vi "superactuator.vi"(8 "error in (no error)":errorcluster, 11 "BMC in":refnum<class "BMC.lvclass">) -> (0 "error out":errorcluster, 3 "BMC out":refnum<class "BMC.lvclass">)   [LabVIEW 2012, in "BMC.lvclass"]
uses:
  BMC.lvclass
  BMC.lvclass/BMC.ctl
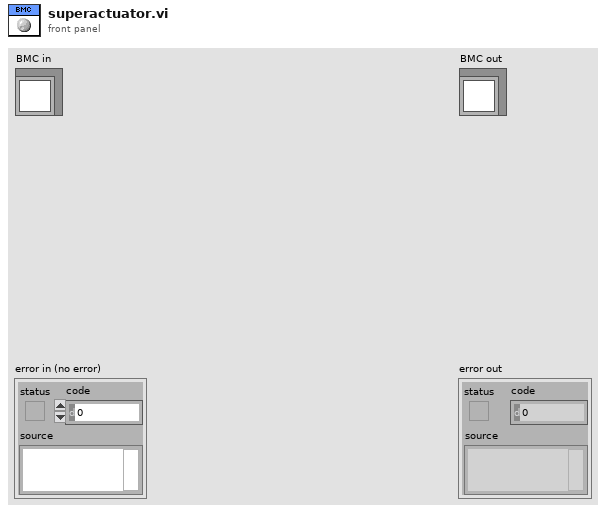
[diagram p1: front panel]
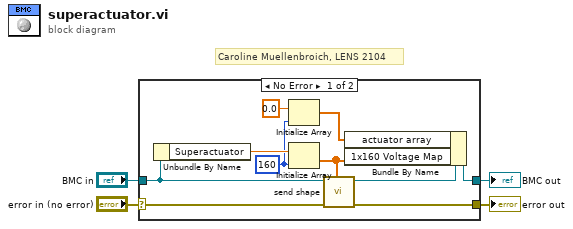
[diagram p0: block diagram]
diagram:
  # "Caroline Muellenbroich, LENS 2104"
  n1 = case shown="No Error" "error in (no error)" {
    selector: "error in (no error)" -> [w13 w16]
    tunnel: [w12 w16] -> w3
    tunnel: [w9 w15] -> w1
    tunnel: "BMC in" -> [w11 w15]
    frame No Error {
      w7 = 160 ("dimension size")
      n2 = Unbundle By Name(w11) -> ("Superactuator"=w14:dbl)
      n3 = Initialize Array(0.0 ("element"), w7) -> (w5:dbl[])
      n4 = Initialize Array(w14, w7) -> (w8:dbl[])
      n5 = call-dynamic "send shape.vi"("error in (no error)"=w13, "1x160 Voltage Map"=w8, "BMC in"=w11) -> ("error out"=w12:errorcluster, "BMC out"=w10:refnum<class "BMC.lvclass">)  [unwired: 7 in]
      n6 = Bundle By Name(cluster=w10, "actuator array"=w5, "1x160 Voltage Map"=w8) -> (w9:refnum<class "BMC.lvclass">)
    }
    frame Error {
    }
  }
  "error out" <- w3
  "BMC out" <- w1
